vi "Write LM Read Rate.vi"(8 "error in (no error)":errorcluster, 10 "Fast?":bool, 11 "Level Meter in":refnum<class "Level Meter.lvclass">) -> (0 "error out":errorcluster, 3 "Level Meter out":refnum<class "Level Meter.lvclass">)   [LabVIEW 2023, in "Level Meter.lvclass"]
uses:
  Level Meter.lvclass
  Level Meter.lvclass/Level Meter.ctl
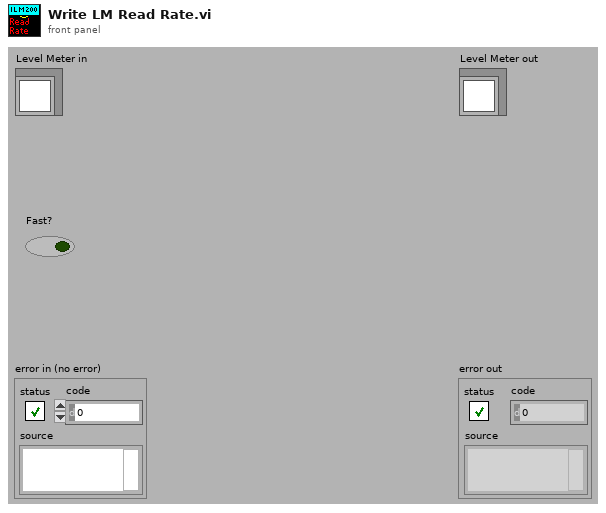
[diagram p1: front panel]
types:
  T1 = typedef "OxfordAddress.ctl" = cluster{"Com Port":i32, "ISOBUS Address":i32, "GPIB Address":i16, "Communication":enum16{"RS232", "ISOBUS", "GPIB", "Gateway"}}
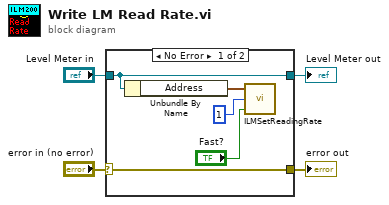
[diagram p0: block diagram]
diagram:
  n1 = case shown="No Error" "error in (no error)" {
    selector: "error in (no error)" -> [w6 w10]
    tunnel: [w6 w10] -> w3
    tunnel: "Level Meter in" -> [w5 w11]
    tunnel: [w5 w11] -> w1
    frame No Error {
      n2 = Unbundle By Name(w5) -> ("Address"=w8:T1)
      n3 = call "ILMSetReadingRate.vi"("Fast"="Fast?", "Channel(1-3)"=1, "Address"=w8) -> ()  [unwired: 1 out]
    }
    frame Error {
    }
  }
  "Level Meter out" <- w1
  "error out" <- w3
